vi "test.vi"() -> ()   [LabVIEW 2010, in "ImageCollection.lvclass"]
uses:
  ImageCollection.lvclass
  storage_mode_enum.ctl
  type_enum.ctl
  saving_parameters_cluster.ctl
  Image/Image/target_format_enum.ctl
  Image/Image/Image.lvclass
  add_mode_enum.ctl
panel:
  in  "saving parameters":T1={"write OME header?"=TRUE, "save as list file?"=FALSE, "force format?"=enum."uint16", "multiplication factor"=1.0, "offset"=0.0}
  in  "getImageByIndexButton":bool
  in  "index":i32
  out "images":T3[](array[plugin-control])
  in  "depth":dbl[unit]
  out "type":T4
  out "total z depth":dbl[unit]
  out "movie length":dbl[unit]
  in  "Image Type":T5=7 items=["Grayscale (U8)", "Grayscale (I16)", "Grayscale (SGL)", "Complex (CSG)", "RGB (U32)", "HSL (U32)", "RGB (U64)", "Grayscale (U16)"]
  in  "load button":bool
  out "time stamp":timestamp
  in  "interval":dbl[unit]
  in  "merge time intervals":bool
  in  "save via ImageJ":bool
  in  "divisor":dbl
  in  "divide":bool
  in  "factor":dbl
  in  "multiply":bool
  in  "all?":bool
  in  "all images?":bool
  out "difference":dbl[unit]
  in  "relative time":dbl[unit]
  in  "get image":bool
  out "current number of images":i32
  in  "storage mode":T6
  in  "range":i32=1 min=1
  in  "first index":i32 min=0
  in  "delete":bool
  in  "duplicate":bool
  in  "bunch size":i32=1 min=1
  in  "merge":bool
  in  "range":i32=1 min=1
  in  "first index":i32 min=0
  in  "calculate average":bool
  out "result":T3(plugin-control)
  in  "add image":bool
  in  "stop":bool
  out "error out":errorcluster
  # "or"
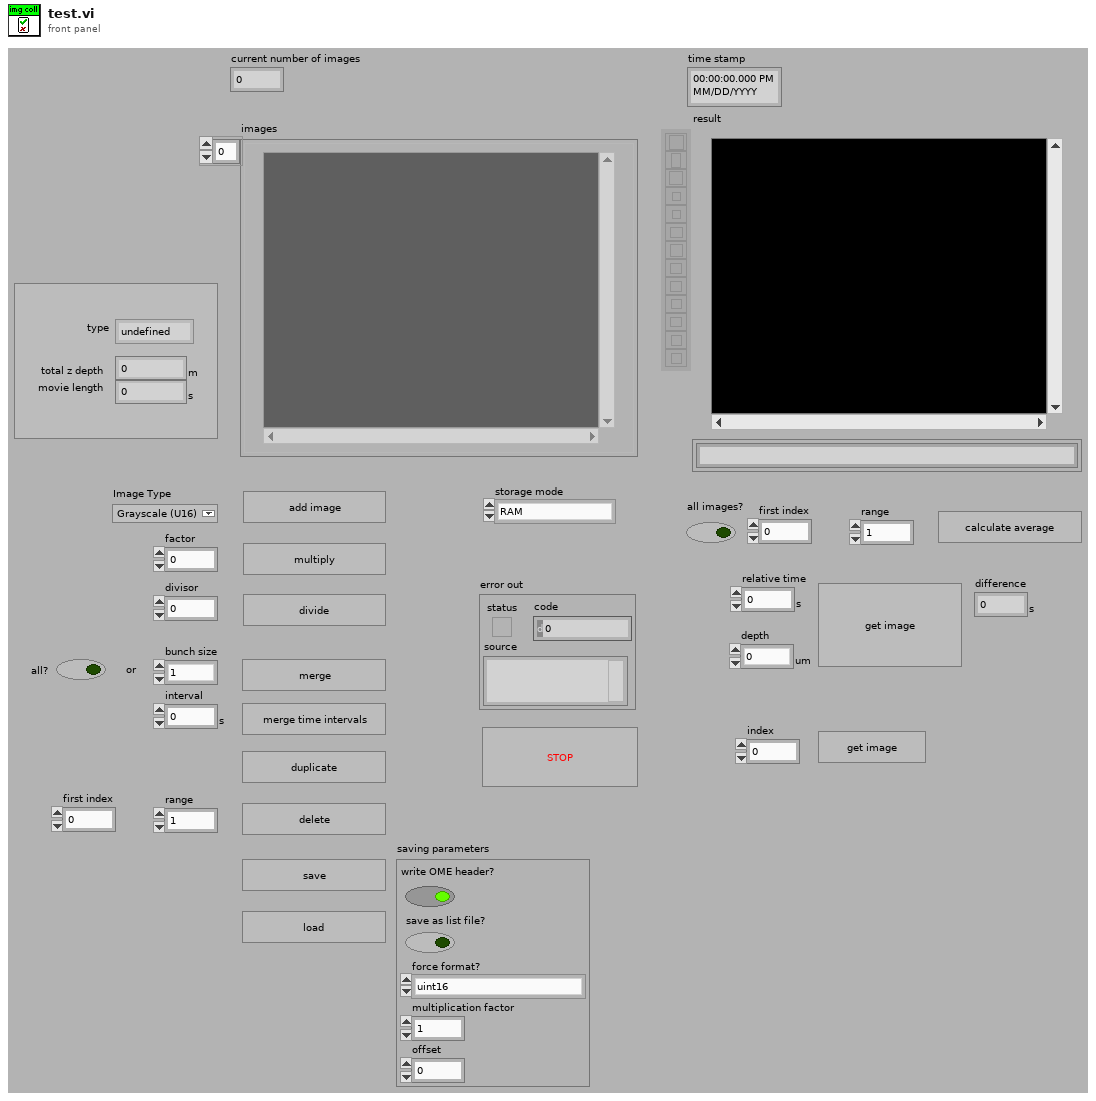
[diagram p1: front panel]
types:
  T1 = typedef "ImageCollection.lvclass/saving_parameters_cluster.ctl" = cluster{"write OME header?":bool, "save as list file?":bool, "force format?":T2, "multiplication factor":dbl, "offset":dbl}
  T2 = typedef "target_format_enum.ctl" = enum16{"don't force", "uint8", "uint16", "int16", "uint32", "int32", "single float"}
  T3 = typedef "IMAQ Image.ctl" = refnum<image>
  T4 = typedef "type_enum.ctl" = enum16{"undefined", "movie", "z-stack"}
  T5 = typedef "Image Type" = u32
  T6 = typedef "ImageCollection.lvclass/storage_mode_enum.ctl" = enum16{"RAM", "single files", "multipage TIFF (read-only)"}
  T7 = typedef "ImageCollection.lvclass/add_mode_enum.ctl" = enum16{"instance", "copy"}
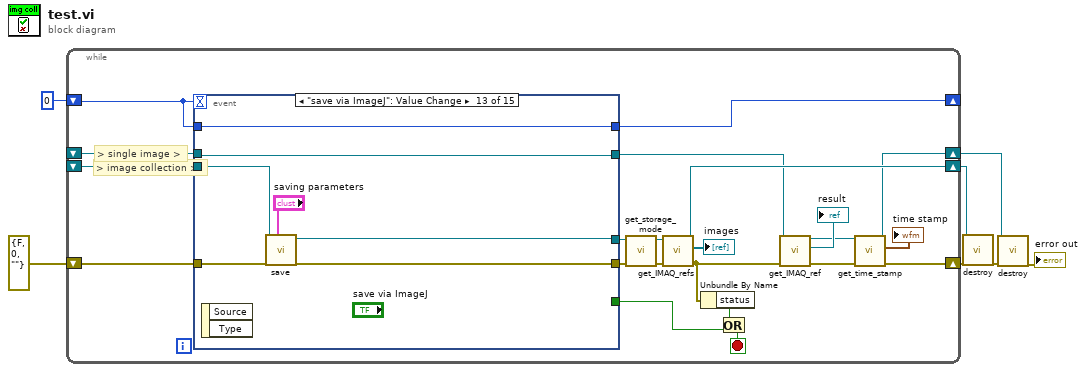
[diagram p0: block diagram]
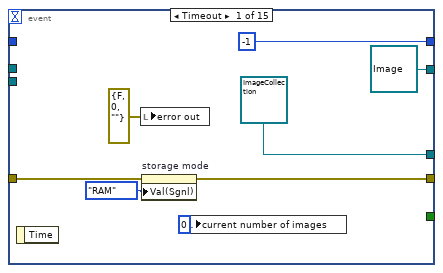
[diagram p2: hidden frame]
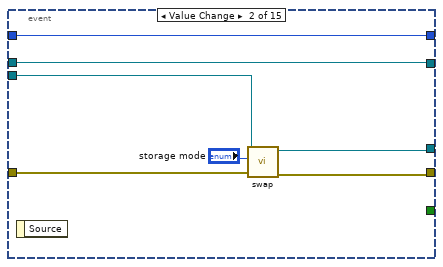
[diagram p3: hidden frame]
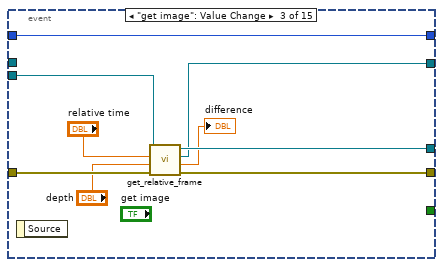
[diagram p4: hidden frame]
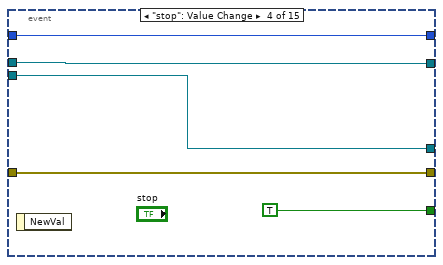
[diagram p5: hidden frame]
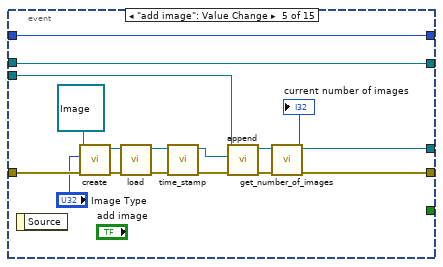
[diagram p6: hidden frame]
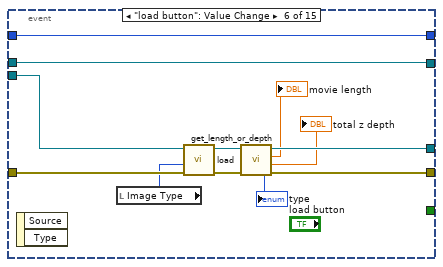
[diagram p7: hidden frame]
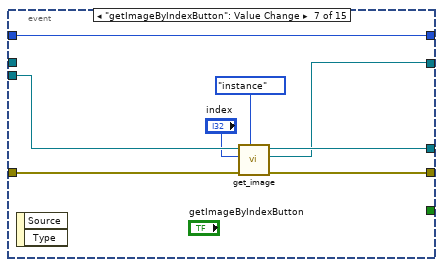
[diagram p8: hidden frame]
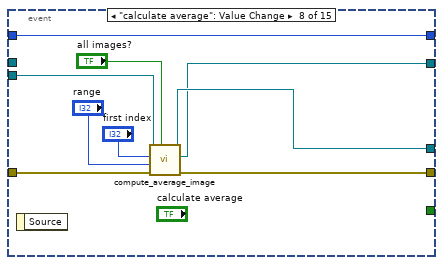
[diagram p9: hidden frame]
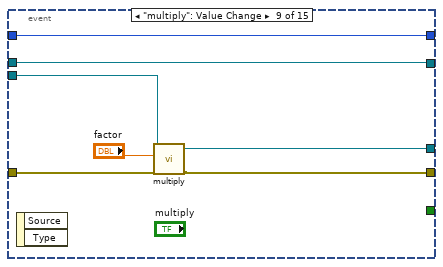
[diagram p10: hidden frame]
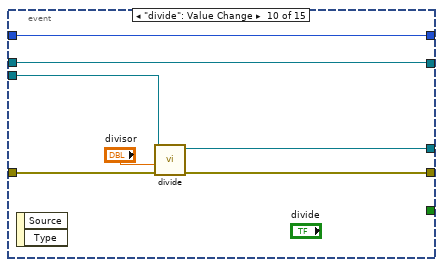
[diagram p11: hidden frame]
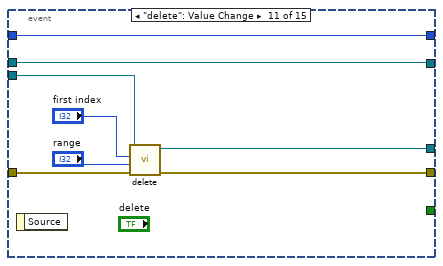
[diagram p12: hidden frame]
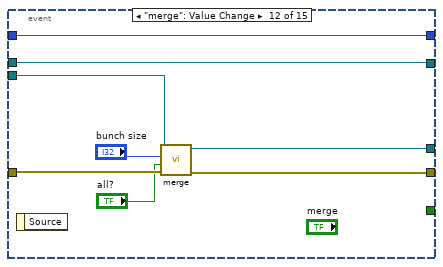
[diagram p13: hidden frame]
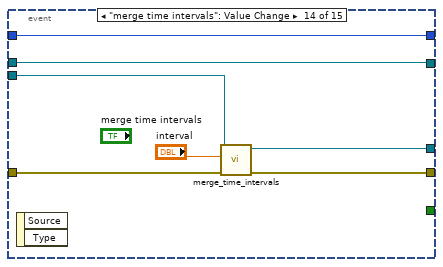
[diagram p14: hidden frame]
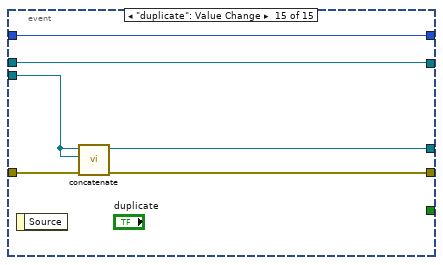
[diagram p15: hidden frame]
diagram:
  n1 = while {
    shift-right: [w28] -> _
    shift-left: 0 -> [w29]
    shift-right: [w17] -> w4
    shift-left: _ -> [w26]
    shift-right: [w11] -> w1
    shift-left: _ -> [w22]
    shift-right: [w10] -> w5
    shift-left: errorcluster {"status"=FALSE, "code"=0, "source"=""} ("error out") -> [w27]
    stop <- w23 stop-if-true
    # "> image collection >"
    # "> single image >"
    n2 = event shown="[12] \"save via ImageJ\": Value Change" {
      selector: _ -> [_ _ _ _ _ _ _ _ _ _ _ _ _ _ _]
      dyn-events: _ -> [_ _ _ _ _ _ _ _ _ _ _ _ _ _ _]
      timeout: w29 -> [_ _ _ _ _ _ _ _ _ _ _ _ _ _ _]
      tunnel: w29 -> [_ w39 w53 w57 w75 w87 w95 w103 w105 w118 w123 w129 w141 w148 w149]
      tunnel: [-1 w39 w53 w57 w75 w87 w95 w103 w105 w118 w123 w129 w141 w148 w149] -> w28
      tunnel: w27 -> [w36 w44 w52 w56 w73 w85 w94 w104 w111 w116 w126 w133 w139 w144 w154]
      tunnel: [_ _ _ TRUE _ _ _ _ _ _ _ _ _ _ _] -> w24
      tunnel: [w30 w43 w48 w56 w65 w82 w93 w97 w110 w115 w125 w128 w136 w143 w152] -> w21
      tunnel: [refnum<class "ImageCollection.lvclass"> refnum ("ImageCollection.lvclass") w40 w49 w55 w67 w80 w91 w99 w107 w114 w121 w130 w137 w145 w150] -> w20
      tunnel: w26 -> [_ w41 w50 w55 w74 w84 w92 w100 w109 w113 w122 w132 w138 w146 w151]
      tunnel: [refnum<class "Image.lvclass"> refnum ("Image.lvclass out") w42 w46 w54 w69 w86 w90 w98 w106 w117 w124 w134 w140 w147 w153] -> w15
      tunnel: w22 -> [_ w42 _ w54 w69 w86 _ _ w106 w117 w124 w134 w140 w147 w153]
      event Timeout {
        n3 = event-data() -> ()  [unwired: 2 out]
        n4 = local write "error out"(errorcluster {"status"=FALSE, "code"=0, "source"=""} ("error out")) -> ()
        n5 = property on="storage mode" class="Enum (strict)"(error in=w36, "Val(Sgnl)"=enum16{"RAM", "single files"}."RAM" ("Value (Signaling)")) -> (error out=w30:errorcluster)  [unwired: 1 in, 1 out]
        n6 = local write "current number of images"(0 ("current number of images")) -> ()
      }
      event Value Change {
        n7 = event-data() -> ()  [unwired: 2 out]
        n8 = call-dynamic "swap.vi"("error in (no error)"=w44, "target storage mode"="storage mode", "ImageCollection in"=w41) -> ("error out"=w43:errorcluster, "ImageCollection out"=w40:refnum<class "ImageCollection.lvclass">)  [unwired: 7 out]
      }
      event "get image": Value Change {
        n9 = event-data() -> ()  [unwired: 2 out]
        n10 = call-dynamic "get_relative_frame.vi"("error in (no error)"=w52, "relative depth"="depth", "relative time"="relative time", "ImageCollection in"=w50) -> ("error out"=w48:errorcluster, "difference"=→"difference":dbl[unit], "frame"=w46:refnum<class "Image.lvclass">, "ImageCollection out"=w49:refnum<class "ImageCollection.lvclass">)  [unwired: 4 out]
      }
      event "stop": Value Change {
        n11 = event-data() -> ()  [unwired: 2 out]
      }
      event "add image": Value Change {
        n12 = event-data() -> ()  [unwired: 2 out]
        n13 = call "create.vi"("error in (no error)"=w73, "Image Type"="Image Type", "Image in"=refnum<class "Image.lvclass"> refnum ("Image.lvclass")) -> ("error out"=w72:errorcluster, "Image out"=w71:refnum<class "Image.lvclass">)  [unwired: 1 in, 6 out]
        n14 = call-dynamic "load.vi"("error in (no error)"=w72, "Image in"=w71) -> ("error out"=w63:errorcluster, "Image out"=w62:refnum<class "Image.lvclass">)  [unwired: 2 in, 6 out]
        n15 = call-dynamic "time_stamp.vi"("error in (no error)"=w63, "Image in"=w62) -> ("error out"=w60:errorcluster, "Image out"=w61:refnum<class "Image.lvclass">)  [unwired: 8 out]
        n16 = call-dynamic "append.vi"("error in (no error)"=w60, "Image.lvclass"=w61, "ImageCollection in"=w74) -> ("error out"=w66:errorcluster, "ImageCollection out"=w68:refnum<class "ImageCollection.lvclass">)  [unwired: 1 in, 6 out]
        n17 = call-dynamic "get_number_of_images.vi"("error in (no error)"=w66, "ImageCollection in"=w68) -> ("error out"=w65:errorcluster, "size"=→"current number of images":i32, "ImageCollection out"=w67:refnum<class "ImageCollection.lvclass">)  [unwired: 7 out]
      }
      event "load button": Value Change {
        n18 = event-data() -> ()  [unwired: 3 out]
        n19 = local read "Image Type"() -> (w76:T5)
        n20 = call "load.vi"("error in (no error)"=w85, "Image Type"=w76, "ImageCollection in"=w84) -> ("error out"=w83:errorcluster, "ImageCollection out"=w81:refnum<class "ImageCollection.lvclass">)  [unwired: 4 in, 3 out]
        n21 = call "get_length_or_depth.vi"("error in (no error)"=w83, "ImageCollection in"=w81) -> ("error out"=w82:errorcluster, "total z depth"=→"total z depth":dbl[unit], "movie length"=→"movie length":dbl[unit], "ImageCollection out"=w80:refnum<class "ImageCollection.lvclass">, "type"=→"type":T4)  [unwired: 5 in]
      }
      event "getImageByIndexButton": Value Change {
        n22 = event-data() -> ()  [unwired: 3 out]
        n23 = call-dynamic "get_image.vi"("get image as..."=add_mode_enum."instance", "error in (no error)"=w94, "index"="index", "ImageCollection in"=w92) -> ("error out"=w93:errorcluster, "Image.lvclass"=w90:refnum<class "Image.lvclass">, "ImageCollection out"=w91:refnum<class "ImageCollection.lvclass">)  [unwired: 5 in]
      }
      event "calculate average": Value Change {
        n24 = event-data() -> ()  [unwired: 2 out]
        n25 = call-dynamic "compute_average_image.vi"("all?"="all images?", "error in (no error)"=w104, "range"="range", "start index"="first index", "ImageCollection in"=w100) -> ("error out"=w97:errorcluster, "averaged image"=w98:refnum<class "Image.lvclass">, "ImageCollection out"=w99:refnum<class "ImageCollection.lvclass">)  [unwired: 4 out]
      }
      event "multiply": Value Change {
        n26 = event-data() -> ()  [unwired: 3 out]
        n27 = call "multiply.vi"("error in (no error)"=w111, "factor"="factor", "ImageCollection in"=w109) -> ("error out"=w110:errorcluster, "ImageCollection out"=w107:refnum<class "ImageCollection.lvclass">)  [unwired: 7 out]
      }
      event "divide": Value Change {
        n28 = event-data() -> ()  [unwired: 3 out]
        n29 = call-dynamic "divide.vi"("error in (no error)"=w116, "divisor"="divisor", "ImageCollection in"=w113) -> ("error out"=w115:errorcluster, "ImageCollection out"=w114:refnum<class "ImageCollection.lvclass">)  [unwired: 1 in, 6 out]
      }
      event "delete": Value Change {
        n30 = event-data() -> ()  [unwired: 2 out]
        n31 = call-dynamic "delete.vi"("error in (no error)"=w126, "range"="range", "start index"="first index", "ImageCollection in"=w122) -> ("error out"=w125:errorcluster, "ImageCollection out"=w121:refnum<class "ImageCollection.lvclass">)  [unwired: 6 out]
      }
      event "merge": Value Change {
        n32 = event-data() -> ()  [unwired: 2 out]
        n33 = call-dynamic "merge.vi"("error in (no error)"=w133, "all?"="all?", "bunch size"="bunch size", "ImageCollection in"=w132) -> ("error out"=w128:errorcluster, "ImageCollection out"=w130:refnum<class "ImageCollection.lvclass">)  [unwired: 6 out]
      }
      event "save via ImageJ": Value Change {
        n34 = event-data() -> ()  [unwired: 3 out]
        n35 = call "save.vi"("saving parameters"="saving parameters", "error in (no error)"=w139, "ImageCollection in"=w138) -> ("error out"=w136:errorcluster, "ImageCollection out"=w137:refnum<class "ImageCollection.lvclass">)  [unwired: 3 in, 4 out]
      }
      event "merge time intervals": Value Change {
        n36 = event-data() -> ()  [unwired: 3 out]
        n37 = call "merge_time_intervals.vi"("error in (no error)"=w144, "merging window size"="interval", "ImageCollection in"=w146) -> ("error out"=w143:errorcluster, "ImageCollection out"=w145:refnum<class "ImageCollection.lvclass">)  [unwired: 7 out]
      }
      event "duplicate": Value Change {
        n38 = event-data() -> ()  [unwired: 2 out]
        n39 = call-dynamic "concatenate.vi"("error in (no error)"=w154, "collection to append"=w151, "ImageCollection in"=w151) -> ("error out"=w152:errorcluster, "ImageCollection out"=w150:refnum<class "ImageCollection.lvclass">)  [unwired: 1 in, 6 out]
      }
    }
    n40 = call-dynamic "get_storage_mode.vi"("error in (no error)"=w21, "ImageCollection.lvclass in"=w20) -> ("error out"=w19:errorcluster, "ImageCollection.lvclass out"=w18:refnum<class "ImageCollection.lvclass">)  [unwired: 8 out]
    n41 = call-dynamic "get_IMAQ_refs.vi"("error in (no error)"=w19, "ImageCollection in"=w18) -> ("error out"=w16:errorcluster, "IMAQ refs"=→"images":T3[], "ImageCollection out"=w17:refnum<class "ImageCollection.lvclass">)  [unwired: 7 out]
    n42 = Unbundle By Name(w16) -> ("status"=w25:bool)
    n43 = Or(x=w25, y=w24) -> (x .or. y?=w23:bool)
    n44 = call-dynamic "get_IMAQ_ref.vi"("error in (no error)"=w16, "Image.lvclass in"=w15) -> ("error out"=w13:errorcluster, "Image"=→"result":T3, "Image.lvclass out"=w12:refnum<class "Image.lvclass">)  [unwired: 7 out]
    n45 = call-dynamic "get_time_stamp.vi"("error in (no error)"=w13, "Image.lvclass in"=w12) -> ("error out"=w10:errorcluster, "timestamp"=→"time stamp":timestamp, "Image.lvclass out"=w11:refnum<class "Image.lvclass">)  [unwired: 7 out]
  }
  n46 = call-dynamic "destroy.vi"("error in (no error)"=w5, "ImageCollection in"=w4) -> ("error out"=w3:errorcluster)  [unwired: 9 out]
  n47 = call-dynamic "destroy.vi"("error in (no error)"=w3, "Image in"=w1) -> ("error out"=→"error out":errorcluster)  [unwired: 9 out]
